vi "Spectrum file name.vi"(10 "Iteracao":i32, 11 "Pasta Destino DESTA aquisicao":path) -> (3 "appended path":path)   [LabVIEW 2021]
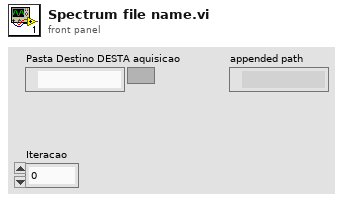
[diagram p1: front panel]
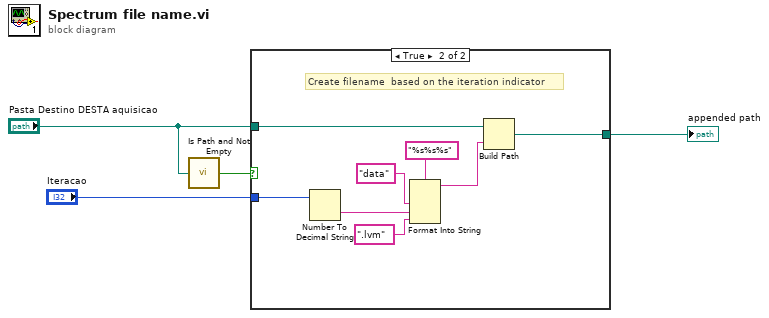
[diagram p0: block diagram]
diagram:
  n1 = call <vilib>:"Is Path and Not Empty.vi"("path"="Pasta Destino DESTA aquisicao") -> ("Is Path and Not Empty?"=w1:bool)  [unwired: 4 in]
  n2 = case shown="True" w1 {
    tunnel: "Iteracao" -> [_ w11]
    tunnel: [_ w9] -> w3
    tunnel: "Pasta Destino DESTA aquisicao" -> [_ w5]
    frame False {
    }
    frame True {
      # "Create filename  based on the iteration indicator"
      n3 = Number To Decimal String(number=w11) -> (decimal integer string=w10:string)  [unwired: 1 in]
      n4 = Format Into String(format string="%s%s%s", "data", w10, ".lvm") -> (resulting string=w8:string)  [unwired: 2 in, 1 out]
      n5 = Build Path(base path=w5, name or relative path=w8) -> (appended path=w9:path)
    }
  }
  "appended path" <- w3
